vi "truncate_string.vi"(11 "String spreadsheet":string) -> (3 "result string":string)   [LabVIEW 2020]
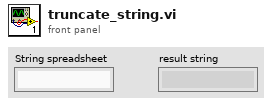
[diagram p1: front panel]
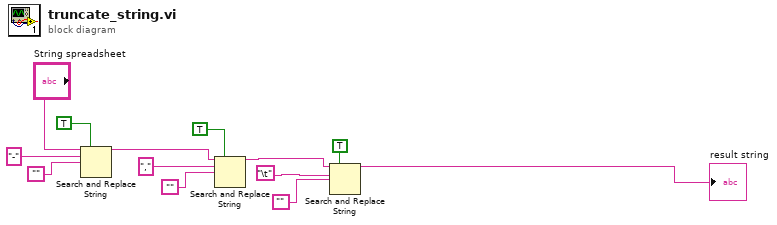
[diagram p0: block diagram]
diagram:
  n1 = Search and Replace String(replace all?=TRUE ("replace all? (F)"), input string="String spreadsheet", search string="-", replace string="") -> (result string=w10:string)  [unwired: 4 in, 3 out]
  n2 = Search and Replace String(replace all?=TRUE ("replace all? (F)"), input string=w10, search string=",", replace string="") -> (result string=w11:string)  [unwired: 4 in, 3 out]
  n3 = Search and Replace String(replace all?=TRUE ("replace all? (F)"), input string=w11, search string="\t", replace string="") -> (result string=→"result string":string)  [unwired: 4 in, 3 out]
